vi "BAM Buffer Connections List.vi"(0 "Connection Cluster":T2, 2 "State":T1=enum."Update", 7 "index":i32, 11 "error in (no error)":errorcluster) -> (4 "Connections":T2[](array[typedef]), 8 "Connection Cluster Out":T2, 15 "error out":errorcluster)   [LabVIEW 2013, in "J1939.lvlib"]
uses:
  J1939.lvlib
  TP/TP Buffer Connection Cluster.ctl
  TP/TP Connections List State.ctl
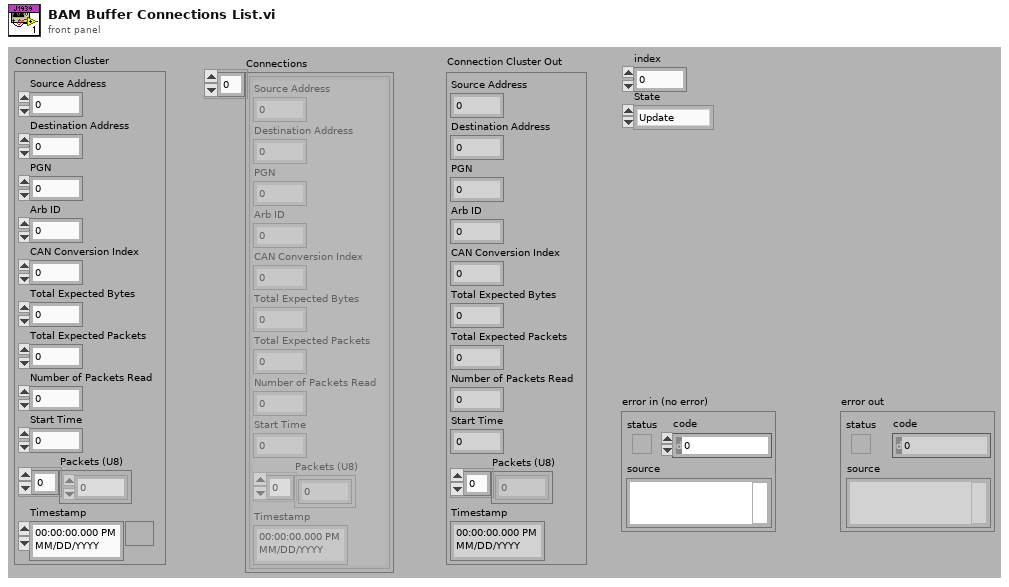
[diagram p1: front panel]
types:
  T1 = typedef "J1939.lvlib/TP Connections List State.ctl" = enum16{"Add", "Update", "Get", "Remove", "Initialize"}
  T2 = typedef "J1939.lvlib/TP Buffer Connection Cluster.ctl" = cluster{"Source Address":u8, "Destination Address":u8, "PGN":u32, "Arb ID":u32, "CAN Conversion Index":u32, "Total Expected Bytes":u16, "Total Expected Packets":u8, "Number of Packets Read":u8, "Start Time":u32, "Packets (U8)":u8[], "Timestamp":timestamp}
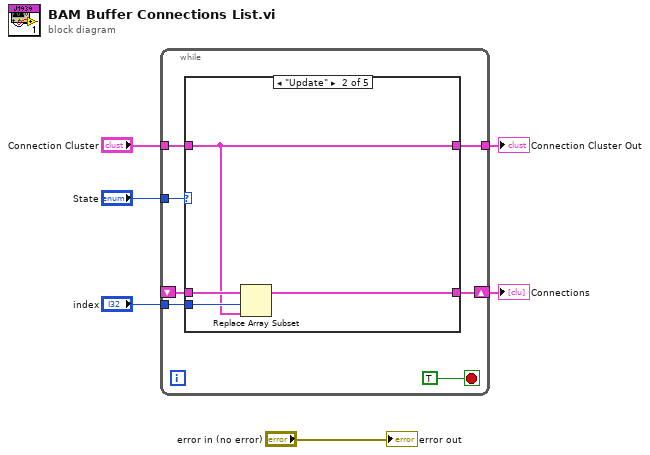
[diagram p0: block diagram]
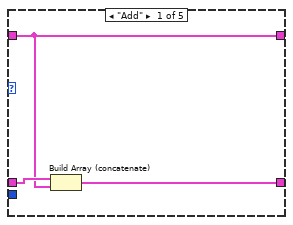
[diagram p2: hidden frame]
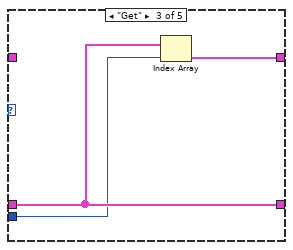
[diagram p3: hidden frame]
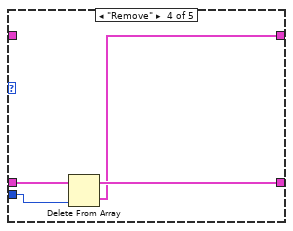
[diagram p4: hidden frame]
diagram:
  n1 = while {
    shift-right: [w10] -> w3
    shift-left: _ -> [w11]
    tunnel: "State" -> [w13]
    tunnel: "Connection Cluster" -> [w12]
    tunnel: "index" -> [w9]
    tunnel: [w8] -> w2
    stop <- TRUE stop-if-true
    n2 = case shown="\"Update\"" w13 {
      tunnel: w12 -> [w14 w18 _ _ _]
      tunnel: w11 -> [w16 w20 w23 w27 _]
      tunnel: [w15 w17 w23 w25 _] -> w10
      tunnel: w9 -> [_ w19 w22 w26 _]
      tunnel: [w14 w18 w21 w24 _] -> w8
      frame "Add" {
        n3 = Build Array (concatenate)(w16, w14) -> (w15:T2[])
      }
      frame "Update" {
        n4 = Replace Array Subset(array=w20, new element=w18, index=w19) -> (w17:T2[])
      }
      frame "Get" {
        n5 = Index Array(array=w23, index=w22) -> (element=w21:T2)
      }
      frame "Remove" {
        n6 = Delete From Array(array=w27, index=w26) -> (deleted portion=w24:T2, array with subset deleted=w25:T2[])  [unwired: 1 in]
      }
      frame "Initialize" {
      }
    }
  }
  "Connection Cluster Out" <- w2
  "Connections" <- w3
  "error out" <- "error in (no error)"
